vi "SetAutoPhase.vi"(5 "error in":T1) -> (19 "error out":T1)   [LabVIEW 2016]
doc: "This VI comes with no input parameter, as it just performs an auto phase."
uses:
  Controls/Error_Out.ctl
  Files_ASC500/DLL/ASC500_RemoteControlV27.dll
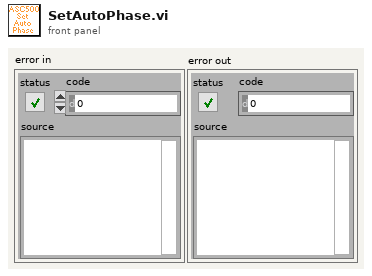
[diagram p1: front panel]
types:
  T1 = typedef "Error_Out.ctl" = errorcluster
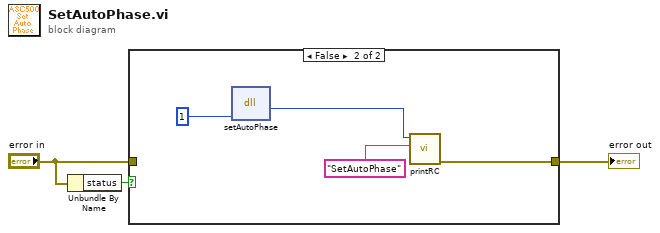
[diagram p0: block diagram]
diagram:
  n1 = Unbundle By Name("error in") -> ("status"=w3:bool)
  n2 = case shown="False" w3 {
    tunnel: [w4 w7] -> w2
    tunnel: "error in" -> [w4 _]
    frame True {
    }
    frame False {
      n3 = dll-call lib="G:/SCMOperations/Share/ELE/Produkt Information/ASC500/04 Remote Control/02 development versions/2018Nov06/Files_ASC500/DLL/ASC500_RemoteControlV27.dll" fn="setAutoPhase"("State"=1) -> ("return type"=w6:i32)  [unwired: 4 in, 2 out]
      n4 = call "printRC.vi"("additional information"="SetAutoPhase", "RC"=w6) -> ("error out"=w7:T1)  [unwired: 9 in]
    }
  }
  "error out" <- w2
